vi "具体消息显示.vi"(2 "error in (no error)":errorcluster caption="错误输入（无错误）", 3 "ID":dbl) -> (0 "error out":errorcluster caption="错误输出", 1 "html_url":string)   [LabVIEW 2012]
panel:
  in  "布尔":bool
  in  "WebBrowser":refnum<k7>(container) caption="网页浏览器"
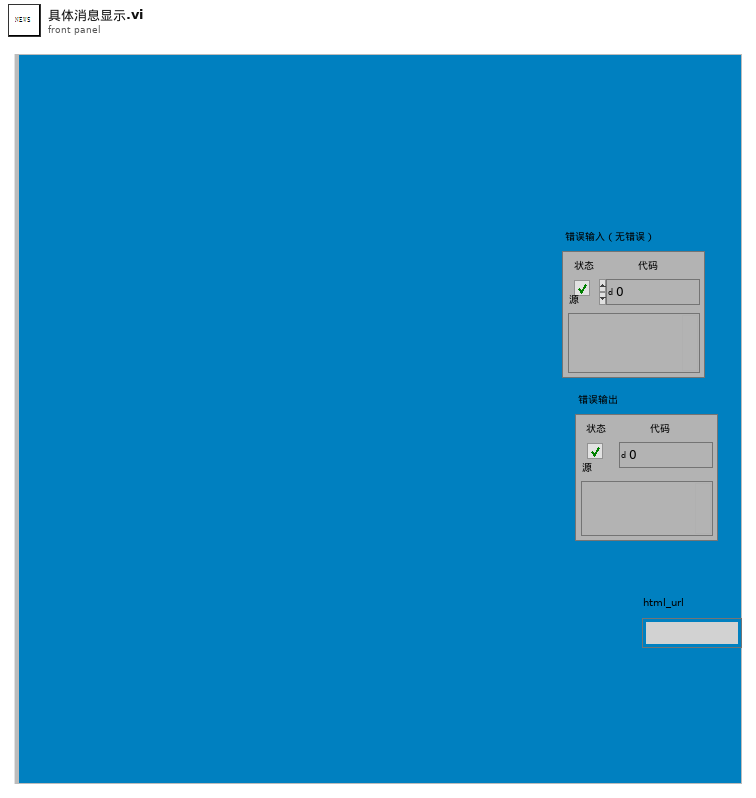
[diagram p1: front panel]
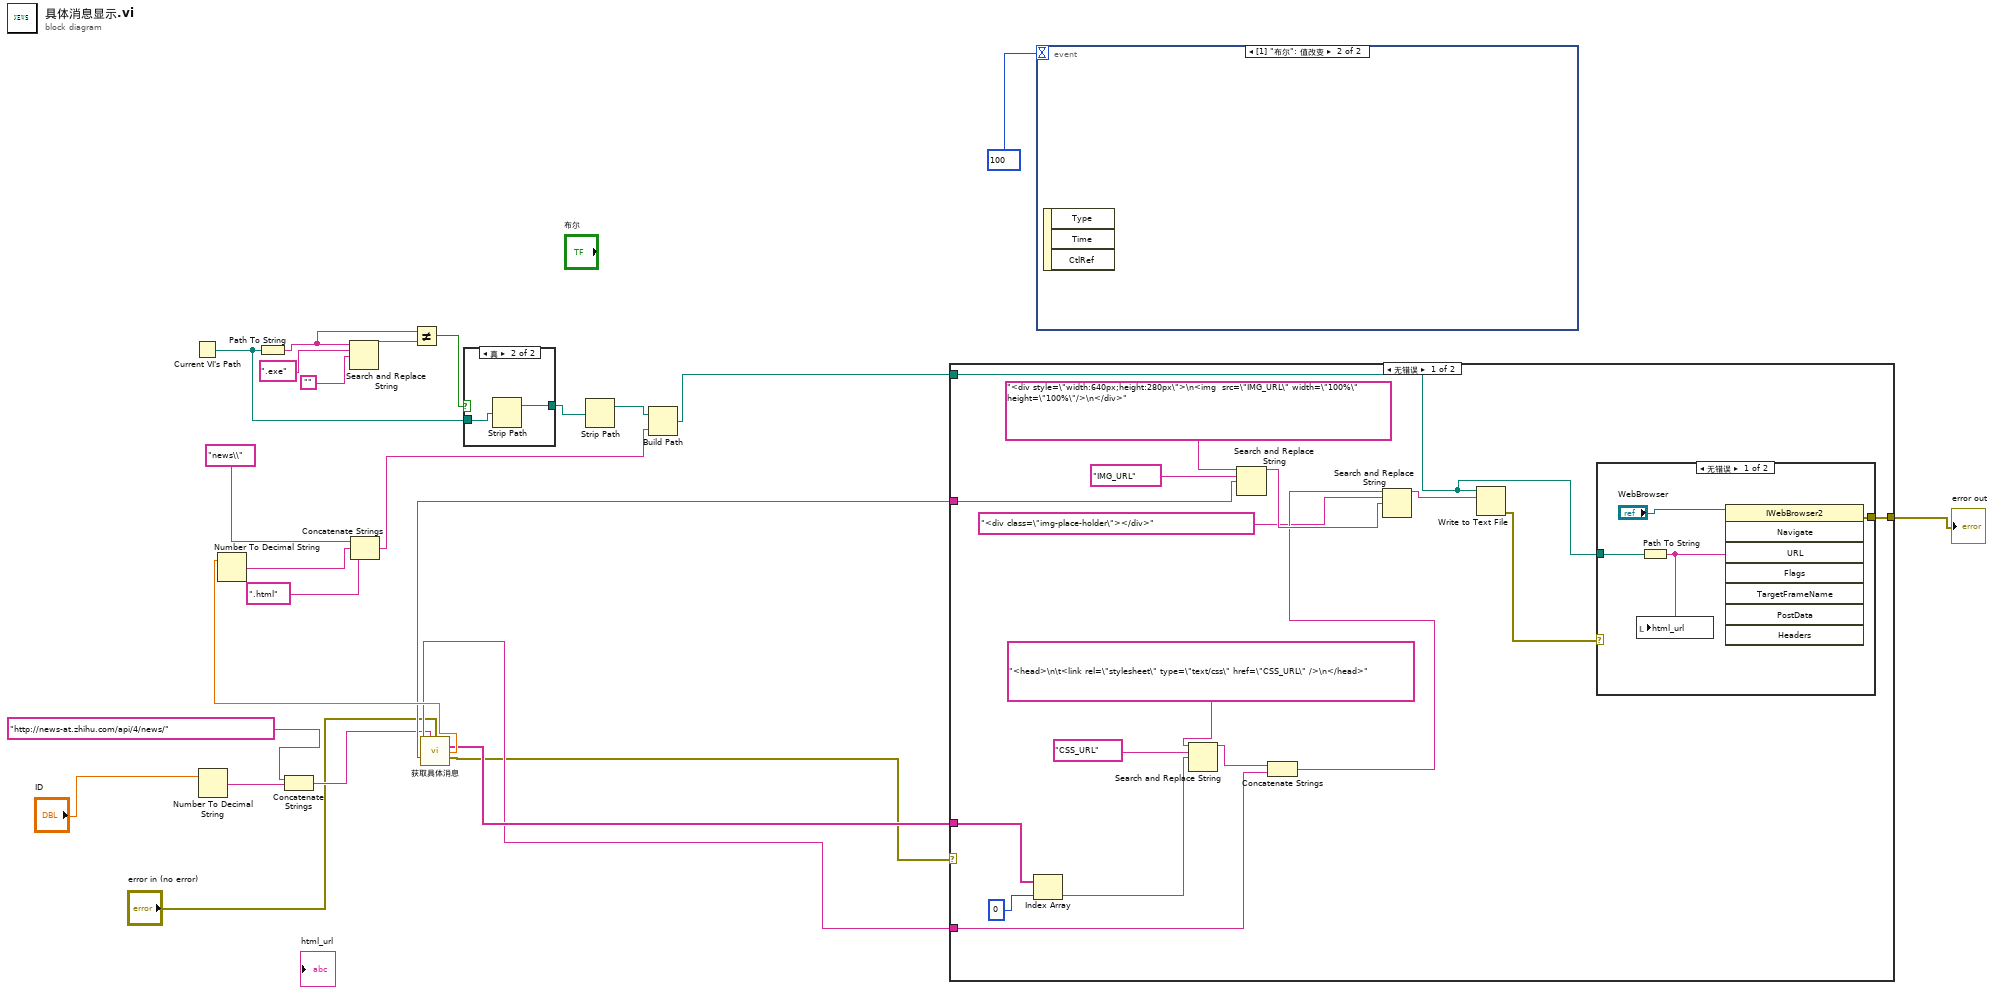
[diagram p0: block diagram]
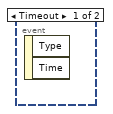
[diagram p3: hidden frame]
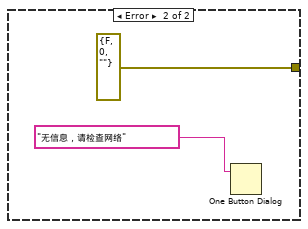
[diagram p4: hidden frame]
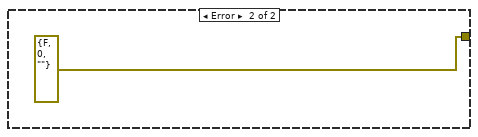
[diagram p5: hidden frame]
diagram:
  n1 = Current VI's Path() -> (path=w21:path)
  n2 = Number To Decimal String(number="ID") -> (decimal integer string=w7:string)  [unwired: 1 in]
  n3 = Path To String(path=w21) -> (string=w19:string)
  n4 = Concatenate Strings("http://news-at.zhihu.com/api/4/news/", w7) -> (w5:string)
  n5 = Search and Replace String(input string=w19, search string=".exe", replace string="") -> (result string=w18:string)  [unwired: 5 in, 3 out]
  n6 = Not Equal?(x=w19, y=w18) -> (x != y?=w20:bool)
  n7 = call "获取具体消息.vi"("URL"=w5, "error in (no error)"="error in (no error)") -> ("body"=w10:string, "css"=w11:string[], "id"=w12:dbl, "image"=w9:string, "error out"=w1:errorcluster)  [unwired: 2 in, 7 out]
  n8 = Number To Decimal String(number=w12) -> (decimal integer string=w13:string)  [unwired: 1 in]
  n9 = Concatenate Strings("news\\", w13, ".html") -> (w24:string)
  n10 = case shown="真" w20 {
    tunnel: w21 -> [w26 w28]
    tunnel: [w26 w27] -> w22
    frame False {
    }
    frame True {
      n11 = Strip Path(path=w28) -> (stripped path=w27:path)  [unwired: 1 out]
    }
  }
  n12 = Strip Path(path=w22) -> (stripped path=w23:path)  [unwired: 1 out]
  n13 = Build Path(base path=w23, name or relative path=w24) -> (appended path=w8:path)
  n14 = case shown="无错误" w1 {
    tunnel: w11 -> [w35 _]
    tunnel: w10 -> [w34 _]
    tunnel: w9 -> [w33 _]
    tunnel: w8 -> [w30 _]
    tunnel: [w29 errorcluster {"status"=FALSE, "code"=0, "source"=""} ("错误常量")] -> w3
    frame No Error {
      n15 = Index Array(array=w35, index=0) -> (element=w43:string)
      n16 = Search and Replace String(input string="<head>\n\t<link rel=\"stylesheet\" type=\"text/css\" href=\"CSS_URL\" />\n</head>", search string="CSS_URL", replace string=w43) -> (result string=w41:string)  [unwired: 5 in, 3 out]
      n17 = Search and Replace String(input string="<div style=\"width:640px;height:280px\">\n<img  src=\"IMG_URL\" width=\"100%\" height=\"100%\"/>\n</div>", search string="IMG_URL", replace string=w33) -> (result string=w38:string)  [unwired: 5 in, 3 out]
      n18 = Concatenate Strings(w41, w34) -> (w37:string)
      n19 = Search and Replace String(input string=w37, search string="<div class=\"img-place-holder\"></div>", replace string=w38) -> (result string=w32:string)  [unwired: 5 in, 3 out]
      n20 = Write to Text File(file (use dialog)=w30, text=w32) -> (error out=w31:errorcluster)  [unwired: 2 in, 2 out]
      n21 = case shown="无错误" w31 {
        tunnel: w30 -> [w49 _]
        tunnel: [w48 errorcluster {"status"=FALSE, "code"=0, "source"=""} ("错误常量")] -> w29
        frame No Error {
          n22 = Path To String(path=w49) -> (string=w47:string)
          n23 = local write "html_url"(w47) -> ()
          n24 = invoke class="IWebBrowser2" method="Navigate"(reference="WebBrowser", "URL"=w47) -> (error out=w48:errorcluster)  [unwired: 6 in, 7 out]
        }
        frame Error {
          n25 = One Button Dialog(message="无信息，请检查网络") -> ()  [unwired: 1 in, 1 out]
        }
      }
    }
    frame Error {
    }
  }
  "error out" <- w3
  n26 = event shown="[1] \"布尔\": 值改变" {
    selector: _ -> [_ _]
    dyn-events: _ -> [_ _]
    timeout: 100 -> [_ _]
    event Timeout {
      n27 = event-data() -> ()  [unwired: 1 in, 2 out]
    }
    event "布尔": Value Change {
      n28 = event-data() -> ()  [unwired: 1 in, 3 out]
    }
  }
